vi "Workspace.UI.DisableState.Set.vi"(8 "error in (no error)":errorcluster, 10 "Enable?":bool=TRUE, 11 "UI.Refs":T1) -> (0 "error out":errorcluster, 3 "UI.Refs out":T1)   [LabVIEW 2019, in "J1939 Workspace Shared.lvlib"]
uses:
  J1939 Workspace Shared.lvlib
  Types/UI.Refs.ctl
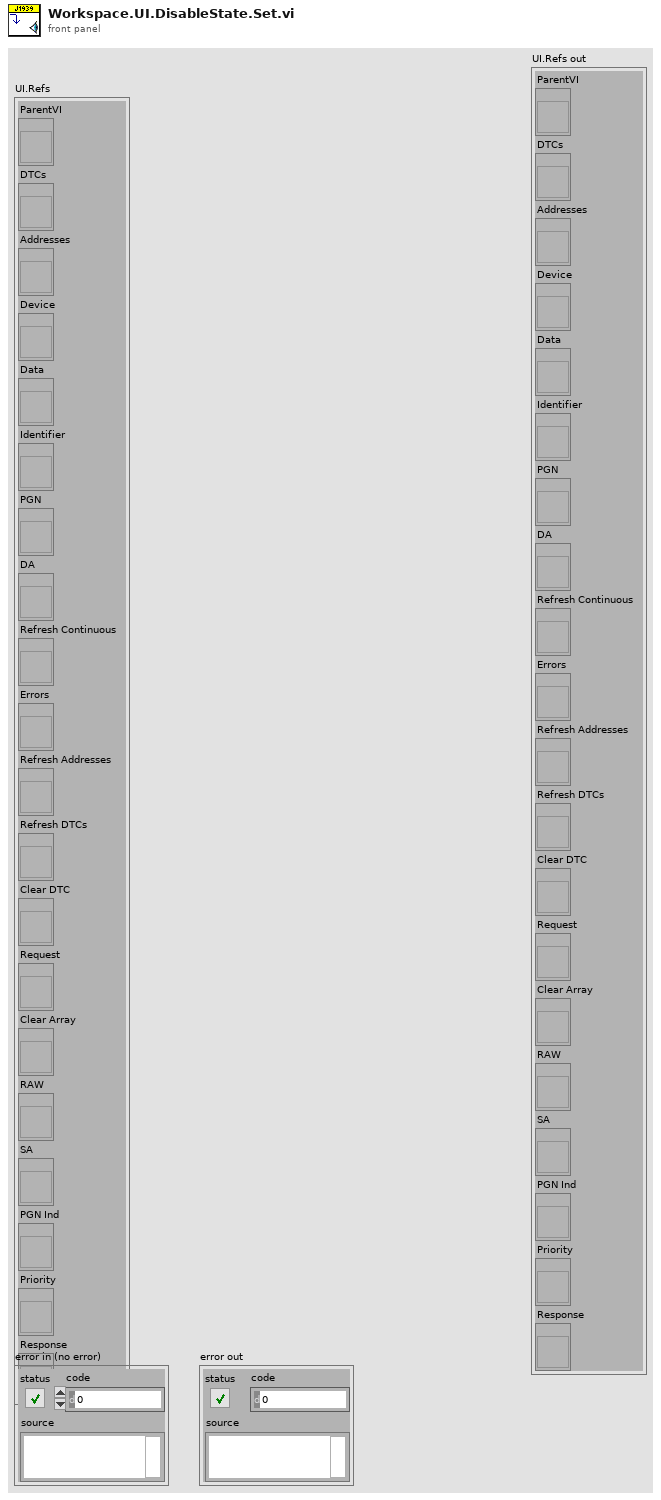
[diagram p1: front panel]
types:
  T1 = typedef "J1939 Workspace Shared.lvlib/UI.Refs.ctl" = cluster{"ParentVI":refnum<vi>, "DTCs":refnum<vi>, "Addresses":refnum<vi>, "Device":refnum<vi>, "Data":refnum<vi>, "Identifier":refnum<vi>, "PGN":refnum<vi>, "DA":refnum<vi>, "Refresh Continuous":refnum<vi>, "Errors":refnum<vi>, "Refresh Addresses":refnum<vi>, "Refresh DTCs":refnum<vi>, "Clear DTC":refnum<vi>, "Request":refnum<vi>, "Clear Array":refnum<vi>, "RAW":refnum<vi>, "SA":refnum<vi>, "PGN Ind":refnum<vi>, "Priority":refnum<vi>, "Response":refnum<vi>}
  T2 = enum8{"Enabled", "Disabled", "Disabled and Grayed Out"}
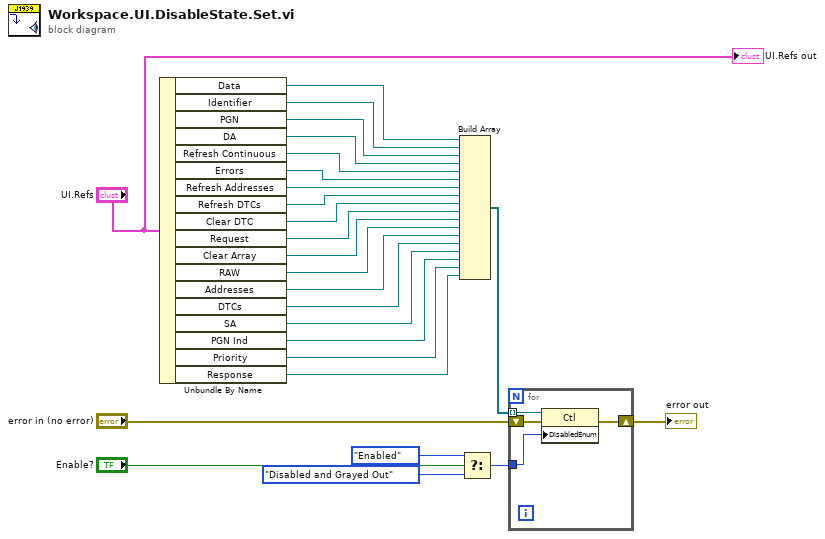
[diagram p0: block diagram]
diagram:
  n1 = Unbundle By Name("UI.Refs") -> ("Data"=w5:refnum<vi>, "Identifier"=w6:refnum<vi>, "PGN"=w7:refnum<vi>, "DA"=w8:refnum<vi>, "Refresh Continuous"=w9:refnum<vi>, "Errors"=w10:refnum<vi>, "Refresh Addresses"=w11:refnum<vi>, "Refresh DTCs"=w12:refnum<vi>, "Clear DTC"=w13:refnum<vi>, "Request"=w14:refnum<vi>, "Clear Array"=w15:refnum<vi>, "RAW"=w16:refnum<vi>, "Addresses"=w20:refnum<vi>, "DTCs"=w21:refnum<vi>, "SA"=w4:refnum<vi>, "PGN Ind"=w3:refnum<vi>, "Priority"=w2:refnum<vi>, "Response"=w1:refnum<vi>)
  n2 = Build Array(w5, w6, w7, w8, w9, w10, w11, w12, w13, w14, w15, w16, w20, w21, w4, w3, w2, w1) -> (w18:refnum<vi>[])
  n3 = Select(t=T2."Enabled" ("Disabled"), s="Enable?", f=T2."Disabled and Grayed Out" ("Disabled")) -> (s? t:f=w25:T2)
  n4 = for {
    shift-right: [w28] -> w19
    shift-left: "error in (no error)" -> [w30]
    tunnel: w18 -> [w29] mode=indexing
    tunnel: w25 -> [w27]
    n5 = property class="Ctl"(reference=w29, error in=w30, "DisabledEnum"=w27) -> (error out=w28:errorcluster)  [unwired: 1 out]
  }
  "error out" <- w19
  "UI.Refs out" <- "UI.Refs"
